vi "Ref_PW_cntr.vi"(0 "Set SN":refnum<vi>, 1 "I Max OFF Time":refnum<vi>, 2 "save flash":refnum<vi>, 3 "Init":bool, 4 "Set Channel Params":refnum<vi>, 5 "BackToBootloader":refnum<vi>, 6 "Set System Params":refnum<vi>, 7 "Clear Log":refnum<vi>, 8 "SetOffsetParam":refnum<vi>, 9 "Tech.Data Ch":refnum<vi>, 10 "I Max Threshold":refnum<vi>, 11 "Config. mode":refnum<vi>, 12 "Set SN":refnum<vi>, 13 "Sys Tech.Data S":refnum<vi>) -> (14 "Tech.Data Ch out":refnum<vi>, 16 "Sys Tech.Data S out":refnum<vi>, 17 "Clear Log out":refnum<vi>, 18 "I Max Threshold out":refnum<vi>, 19 "SetOffsetParam out":refnum<vi>, 20 "Set SN out":refnum<vi>, 21 "save flash out":refnum<vi>, 22 "Set Channel Params out":refnum<vi>, 23 "Set System Params out":refnum<vi>, 24 "Config. mode out":refnum<vi>, 25 "I Max OFF Time out":refnum<vi>, 26 "BackToBootloader out":refnum<vi>, 27 "Set SN out":refnum<vi>)   [LabVIEW 2017]
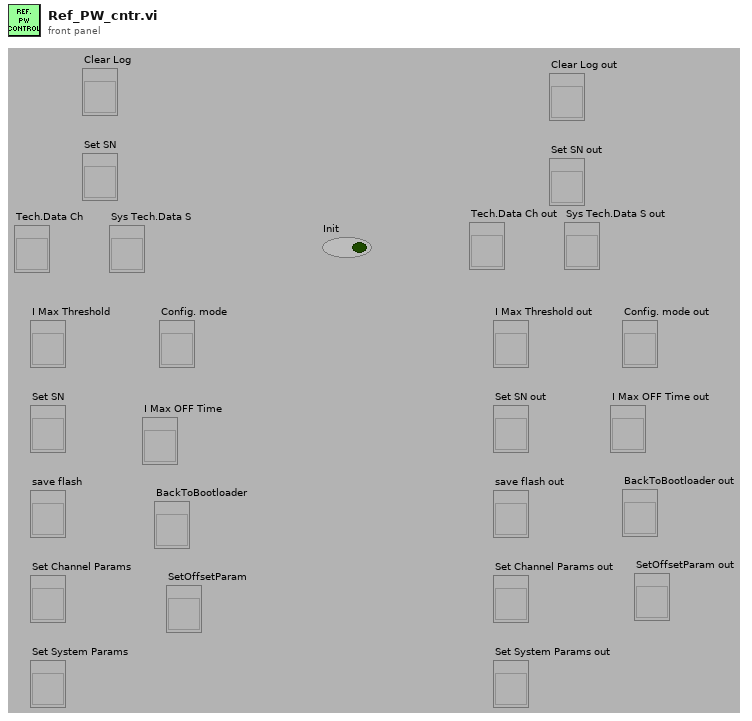
[diagram p1: front panel]
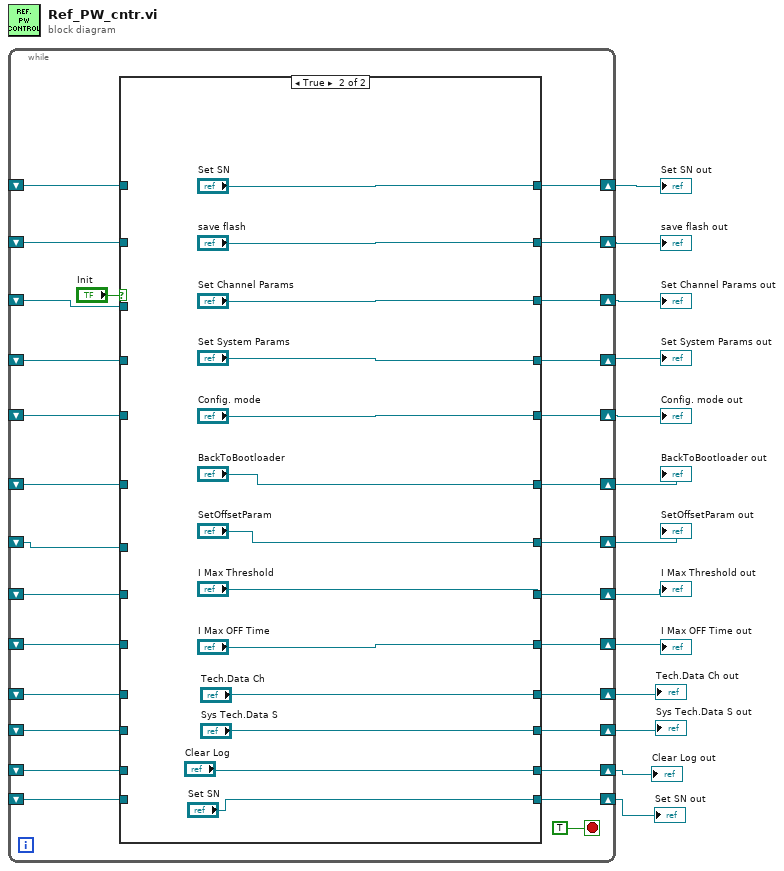
[diagram p0: block diagram]
diagram:
  n1 = while {
    shift-right: [w30] -> w5
    shift-left: _ -> [w36]
    shift-right: [w40] -> w6
    shift-left: _ -> [w35]
    shift-right: [w39] -> w7
    shift-left: _ -> [w34]
    shift-right: [w38] -> w8
    shift-left: _ -> [w33]
    shift-right: [w37] -> w9
    shift-left: _ -> [w32]
    shift-right: [w29] -> w10
    shift-left: _ -> [w28]
    shift-right: [w27] -> w11
    shift-left: _ -> [w26]
    shift-right: [w25] -> w12
    shift-left: _ -> [w19]
    shift-right: [w24] -> w13
    shift-left: _ -> [w18]
    shift-right: [w23] -> w3
    shift-left: _ -> [w17]
    shift-right: [w22] -> w4
    shift-left: _ -> [w16]
    shift-right: [w21] -> w2
    shift-left: _ -> [w15]
    shift-right: [w20] -> w1
    shift-left: _ -> [w14]
    stop <- TRUE stop-if-true
    n2 = case shown="True" "Init" {
      tunnel: [w50 "Set SN"] -> w30
      tunnel: [w54 "save flash"] -> w40
      tunnel: [w53 "Set Channel Params"] -> w39
      tunnel: [w52 "Set System Params"] -> w38
      tunnel: [w51 "Config. mode"] -> w37
      tunnel: w36 -> [w50 _]
      tunnel: w35 -> [w54 _]
      tunnel: w34 -> [w53 _]
      tunnel: w33 -> [w52 _]
      tunnel: w32 -> [w51 _]
      tunnel: [w49 "BackToBootloader"] -> w29
      tunnel: w28 -> [w49 _]
      tunnel: [w48 "SetOffsetParam"] -> w27
      tunnel: w26 -> [w48 _]
      tunnel: [w47 "I Max Threshold"] -> w25
      tunnel: [w46 "I Max OFF Time"] -> w24
      tunnel: [w45 "Tech.Data Ch"] -> w23
      tunnel: [w44 "Sys Tech.Data S"] -> w22
      tunnel: [w43 "Clear Log"] -> w21
      tunnel: [w42 "Set SN"] -> w20
      tunnel: w19 -> [w47 _]
      tunnel: w18 -> [w46 _]
      tunnel: w17 -> [w45 _]
      tunnel: w16 -> [w44 _]
      tunnel: w15 -> [w43 _]
      tunnel: w14 -> [w42 _]
      frame False {
      }
      frame True {
      }
    }
  }
  "Set SN out" <- w5
  "save flash out" <- w6
  "Set Channel Params out" <- w7
  "Set System Params out" <- w8
  "Config. mode out" <- w9
  "BackToBootloader out" <- w10
  "SetOffsetParam out" <- w11
  "I Max Threshold out" <- w12
  "I Max OFF Time out" <- w13
  "Tech.Data Ch out" <- w3
  "Sys Tech.Data S out" <- w4
  "Set SN out" <- w1
  "Clear Log out" <- w2
